vi "sv_Buffer Even-Angle Signal (1 Ch).vi"(0 "initial buffered x[n]":dbl[](array[numeric]), 1 "reset? (True)":bool=TRUE, 5 "even-angle signal":cluster{"r0":dbl, "dr":dbl, "Y":dbl[]}={"r0"=0.0, "dr"=1.0, "Y"=[]} {"r0" format="%.2p"; "dr" format="%.2p"; "Y" format="%.2f"}, 9 "integration cycles":u32) -> (3 "buffered x[n]":dbl[](array[numeric]), 4 "buffered x[n] for analysis":dbl[](array[numeric]), 6 "sample rate":dbl)   [LabVIEW 2017]
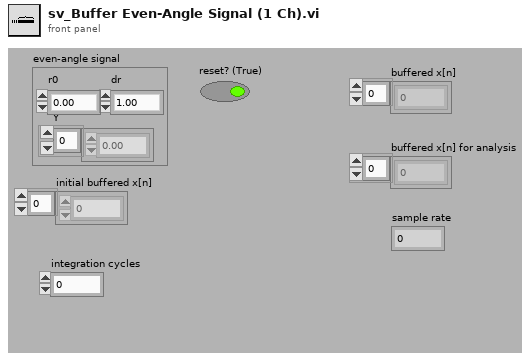
[diagram p1: front panel]
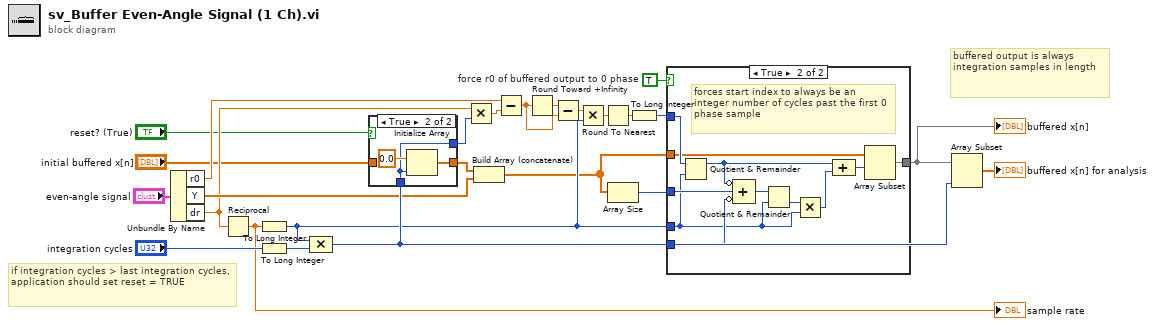
[diagram p0: block diagram]
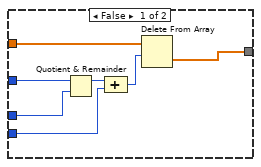
[diagram p2: hidden frame]
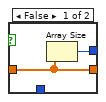
[diagram p3: hidden frame]
diagram:
  w1 = TRUE  # force r0 of buffered output to 0 phase
  # "buffered output is always integration samples in length"
  # "if integration cycles > last integration cycles, application should set reset = TRUE"
  n1 = Unbundle By Name("even-angle signal") -> ("r0"=w17:dbl, "Y"=w21:dbl[], "dr"=w16:dbl)
  n2 = Reciprocal(x=w16) -> (1/x=w15:dbl)
  "sample rate" <- w15
  n3 = To Long Integer(number=w15) -> (32bit integer=w20:i32)
  n4 = To Long Integer(number="integration cycles") -> (32bit integer=w18:i32)
  n5 = Compound Arithmetic op=MULTIPLY(w20, w18) -> (w24:i32)
  n6 = case shown="True" "reset? (True)" {
    tunnel: w24 -> [_ w28]
    tunnel: "initial buffered x[n]" -> [w26 _]
    tunnel: [w26 w29] -> w4
    tunnel: [w27 w28] -> w5
    frame False {
      n7 = Array Size(array=w26) -> (size(s)=w27:i32)
    }
    frame True {
      n8 = Initialize Array(0.0 ("element"), w28) -> (w29:dbl[])
    }
  }
  n9 = Multiply(x=w16, y=w5) -> (x*y=w12:dbl)
  n10 = Build Array (concatenate)(w4, w21) -> (w2:dbl[])
  n11 = Subtract(x=w17, y=w12) -> (x-y=w10:dbl)
  n12 = Round Toward +Infinity(x=w10) -> (ceil(x): smallest int >= x=w11:dbl)
  n13 = Subtract(x=w11, y=w10) -> (x-y=w9:dbl)
  n14 = Multiply(x=w9, y=w20) -> (x*y=w8:dbl)
  n15 = Round To Nearest(number=w8) -> (nearest integer value=w7:dbl)
  n16 = Array Size(array=w2) -> (size(s)=w3:i32)
  n17 = To Long Integer(number=w7) -> (32bit integer=w6:i32)
  n18 = case shown="True" w1 {
    tunnel: w6 -> [_ w48]
    tunnel: w3 -> [w33 w47]
    tunnel: w24 -> [w31 w46]
    tunnel: w2 -> [w35 w41]
    tunnel: [w34 w40] -> w23
    tunnel: w20 -> [w32 w38]
    frame False {
      n19 = Quotient & Remainder(x=w33, y=w32) -> (x-y*floor(x/y)=w36:i32)  [unwired: 1 out]
      n20 = Compound Arithmetic op=ADD(w36, w31) -> (w37:i32)
      n21 = Delete From Array(array=w35, length=w37) -> (deleted portion=w34:dbl[])  [unwired: 1 in, 1 out]
    }
    frame True {
      # "forces start index to always be an integer number of cycles past the first 0 phase sample"
      n22 = Quotient & Remainder(x=w48, y=w38) -> (x-y*floor(x/y)=w42:i32)  [unwired: 1 out]
      n23 = Compound Arithmetic op=ADD(invert w42, w47, invert w46) -> (w45:i32)
      n24 = Quotient & Remainder(x=w45, y=w38) -> (floor(x/y)=w44:i32)  [unwired: 1 out]
      n25 = Multiply(x=w44, y=w38) -> (x*y=w43:i32)
      n26 = Compound Arithmetic op=ADD(w42, w43) -> (w39:i32)
      n27 = Array Subset(array=w41, index=w39) -> (w40:dbl[])  [unwired: 1 in]
    }
  }
  "buffered x[n]" <- w23
  n28 = Array Subset(array=w23, length=w24) -> (→"buffered x[n] for analysis":dbl[])  [unwired: 1 in]
